vi "Check WebSocket Response.vi"(11 "Processing In":refnum<class "Processing.lvclass">) -> (3 "Processing":refnum<class "Processing.lvclass">)   [LabVIEW 2020, in "HTTP Server.lvlib" / "Server.lvclass"]
uses:
  Server.lvclass
  Server.lvclass/Server.ctl
  Processing/Processing.lvclass
  WebSocketUpgradeResponse/WebSocketUpgradeResponse.lvclass
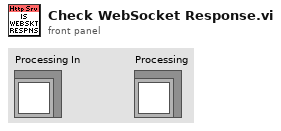
[diagram p1: front panel]
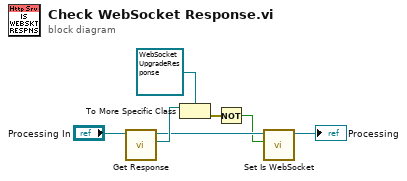
[diagram p0: block diagram]
diagram:
  n1 = call "Get Response.vi"("Processing in"="Processing In") -> ("Response"=w4:refnum<class "Response.lvclass">, "Processing out"=w3:refnum<class "Processing.lvclass">)  [unwired: 9 in]
  n2 = To More Specific Class(target class=refnum<class "WebSocketUpgradeResponse.lvclass"> refnum ("Stream-Websocket.lvlib:WebSocketUpgradeResponse.lvclass"), reference=w4) -> (error out=w6:errorcluster)  [unwired: 1 in, 1 out]
  n3 = Not(x=w6) -> (.not. x?=w1:bool)
  n4 = call "Set Is WebSocket.vi"("Is WebSocket"=w1, "Processing in"=w3) -> ("Processing out"=→"Processing":refnum<class "Processing.lvclass">)  [unwired: 9 in]
